vi "InitConfig.vi"(8 "error control":errorcluster, 11 "configuration file path":path) -> (0 "error indicator":errorcluster, 3 "refnum":T1)   [LabVIEW 2014]
uses:
  <vilib>/Utility/config.llb/Config Data RefNum.ctl
  <vilib>/Utility/config.llb/NI_LVConfig.lvlib
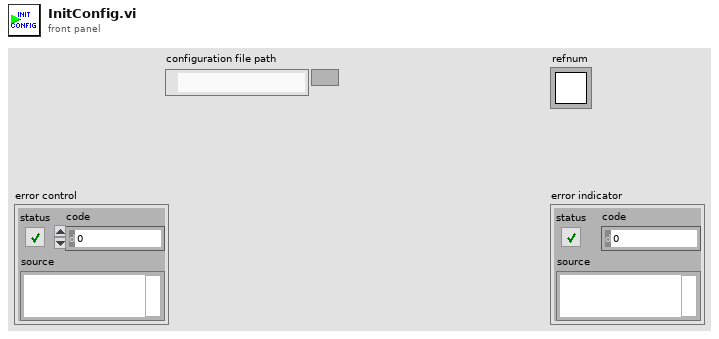
[diagram p1: front panel]
types:
  T1 = typedef "NI_LVConfig.lvlib/Config Data RefNum.ctl" = refnum<k1>
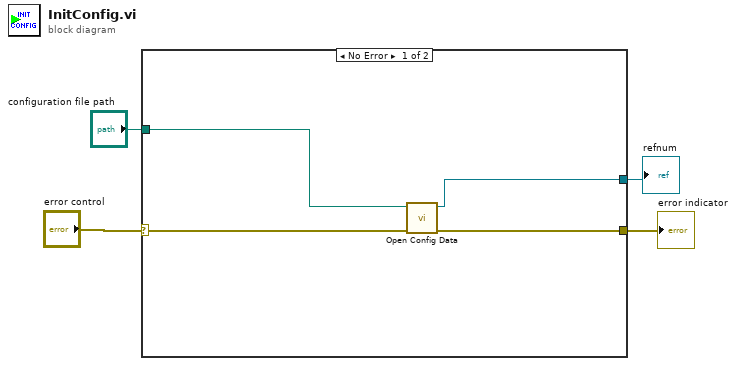
[diagram p0: block diagram]
diagram:
  n1 = case shown="No Error" "error control" {
    selector: "error control" -> [w6 w9]
    tunnel: [w8 w9] -> w3
    tunnel: [w7 _] -> w2
    tunnel: "configuration file path" -> [w5 _]
    frame No Error {
      n2 = call <vilib>:"Open Config Data.vi"("error in (no error)"=w6, "configuration file path"=w5) -> ("error out"=w8:errorcluster, "refnum"=w7:T1)  [unwired: 7 in, 1 out]
    }
    frame Error {
    }
  }
  "error indicator" <- w3
  "refnum" <- w2
